vi "Navigation.vi"(0 "IA State Output in":T1, 7 "a1":dbl=10.0, 9 "a3":dbl=15.0, 11 "GoTo Navigation":bool, 12 "Debug":bool, 13 "output inc":dbl, 14 "output xy":dbl, 15 "output angle":dbl) -> (4 "IA State Output out":T1)   [LabVIEW 2017]
uses:
  Core/AI Input.ctl
  Core/AI Robot.ctl
  Intel/Functions Enum.ctl
  Intel/AttackerStates.ctl
  Path Planning/RRT/PathDests.ctl
  Path Planning/RRT/PathDest.ctl
  Core/AI Ball.ctl
  Core/Field Size.ctl
  Core/AI Judge.ctl
  Intel/Command Enum.ctl
  Util/Events/Events.ctl
panel:
  out "time 10":dbl
  out "time 9":dbl
  out "time 8":dbl
  out "time 7":dbl
  out "time 6":dbl
  out "time 5":dbl
  out "time 4":dbl
  out "time 3":dbl
  out "time 2":dbl
  out "time":dbl
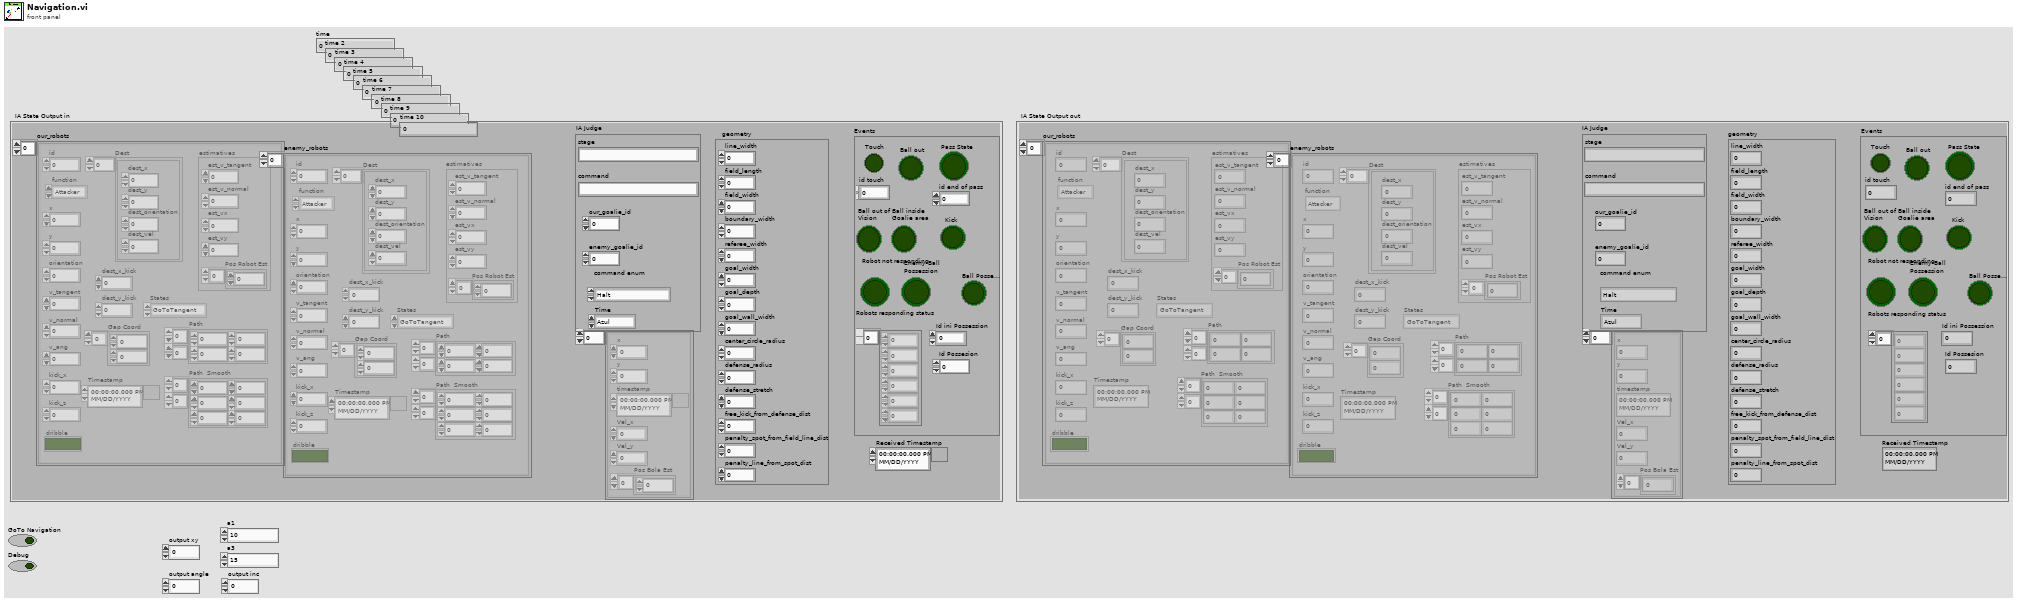
[diagram p1: front panel]
types:
  T1 = typedef "AI Input.ctl" = cluster{"our_robots":T2[], "enemy_robots":T2[], "balls":T7[], "geometry":T8, "IA Judge":T9, "Received Timestamp":timestamp, "Events":T11}
  T2 = typedef "AI Robot.ctl" = cluster{"id":u32, "function":T3, "x":dbl, "y":dbl, "orientation":dbl, "v_tangent":dbl, "v_normal":dbl, "v_ang":dbl, "kick_x":dbl, "kick_z":dbl, "dribble":bool, "Timestamp":timestamp, "estimatives":cluster{"est_v_tangent":dbl, "est_v_normal":dbl, "est_vx":dbl, "est_vy":dbl, "Pos Robot Est":dbl[]}, "dest_x_kick":dbl, "dest_y_kick":dbl, "Gap Coord":dbl[], "States":T4, "Path ":dbl[][], "Path  Smooth":dbl[][], "Dest":T5}
  T3 = typedef "Functions Enum.ctl" = enum16{"Attacker", "Goalie", "Defender", "Striker", "Goto 0", "Dummy", "Kicker", "ZigZag"}
  T4 = typedef "AttackerStates.ctl" = enum16{"Pass", "GoToTangent", "BallGetting", "GoToKick", ""}
  T5 = typedef "PathDests.ctl" = T6[]
  T6 = typedef "PathDest.ctl" = cluster{"dest_x":dbl, "dest_y":dbl, "dest_orientation":dbl, "dest_vel":dbl}
  T7 = typedef "AI Ball.ctl" = cluster{"x":dbl, "y":dbl, "timestamp":timestamp, "Vel_x":dbl, "Vel_y":dbl, "Pos Bola Est":dbl[]}
  T8 = typedef "Field Size.ctl" = cluster{"line_width":u32, "field_length":u32, "field_width":u32, "boundary_width":u32, "referee_width":u32, "goal_width":u32, "goal_depth":u32, "goal_wall_width":u32, "center_circle_radius":u32, "defense_radius":u32, "defense_stretch":u32, "free_kick_from_defense_dist":u32, "penalty_spot_from_field_line_dist":u32, "penalty_line_from_spot_dist":u32}
  T9 = typedef "AI Judge.ctl" = cluster{"stage":string, "command":string, "our_goalie_id":dbl, "enemy_goalie_id":dbl, "command enum":T10, "Time":enum16{"Azul", "Amarelo"}}
  T10 = typedef "Command Enum.ctl" = enum16{"Halt", "Stop", "Force Start", "PKA Normal Start", "Prepare Kickoff Ally", "PKE Normal Start", "Prepare Kickoff Enemy", "Prepare Penalty Ally", "PPA Normal Start", "Prepare Penalty Enemy", "PPE Normal Start", "Direct Free Enemy", "Direct Free Ally", "Indirect Free Enemy", "Indirect Free Ally", "Timeout Enemy", "Timeout Ally", "Goal Enemy", "Goal Ally", "Ball Placement Enemy", "Ball Placement Ally", "Normal Half Time", "Extra Time Break", "Extra Half Time", "None", "Post Game"}
  T11 = typedef "Events.ctl" = cluster{"Touch":bool, "Ball out":bool, "id touch":dbl, "Ball out of \nVision":bool, "Ball inside \nGoalie area":bool, "Robot not responding":bool, "Robots responding status":dbl[], "Enemy Ball \nPossession":bool, "Pass State":bool, "id end of pass":dbl, "Kick":bool, "Id ini Possession":dbl, "Ball Possesion":bool, "Id Possesion":dbl}
  T12 = cluster{"est_v_tangent":dbl, "est_v_normal":dbl, "est_vx":dbl, "est_vy":dbl, "Pos Robot Est":dbl[]}
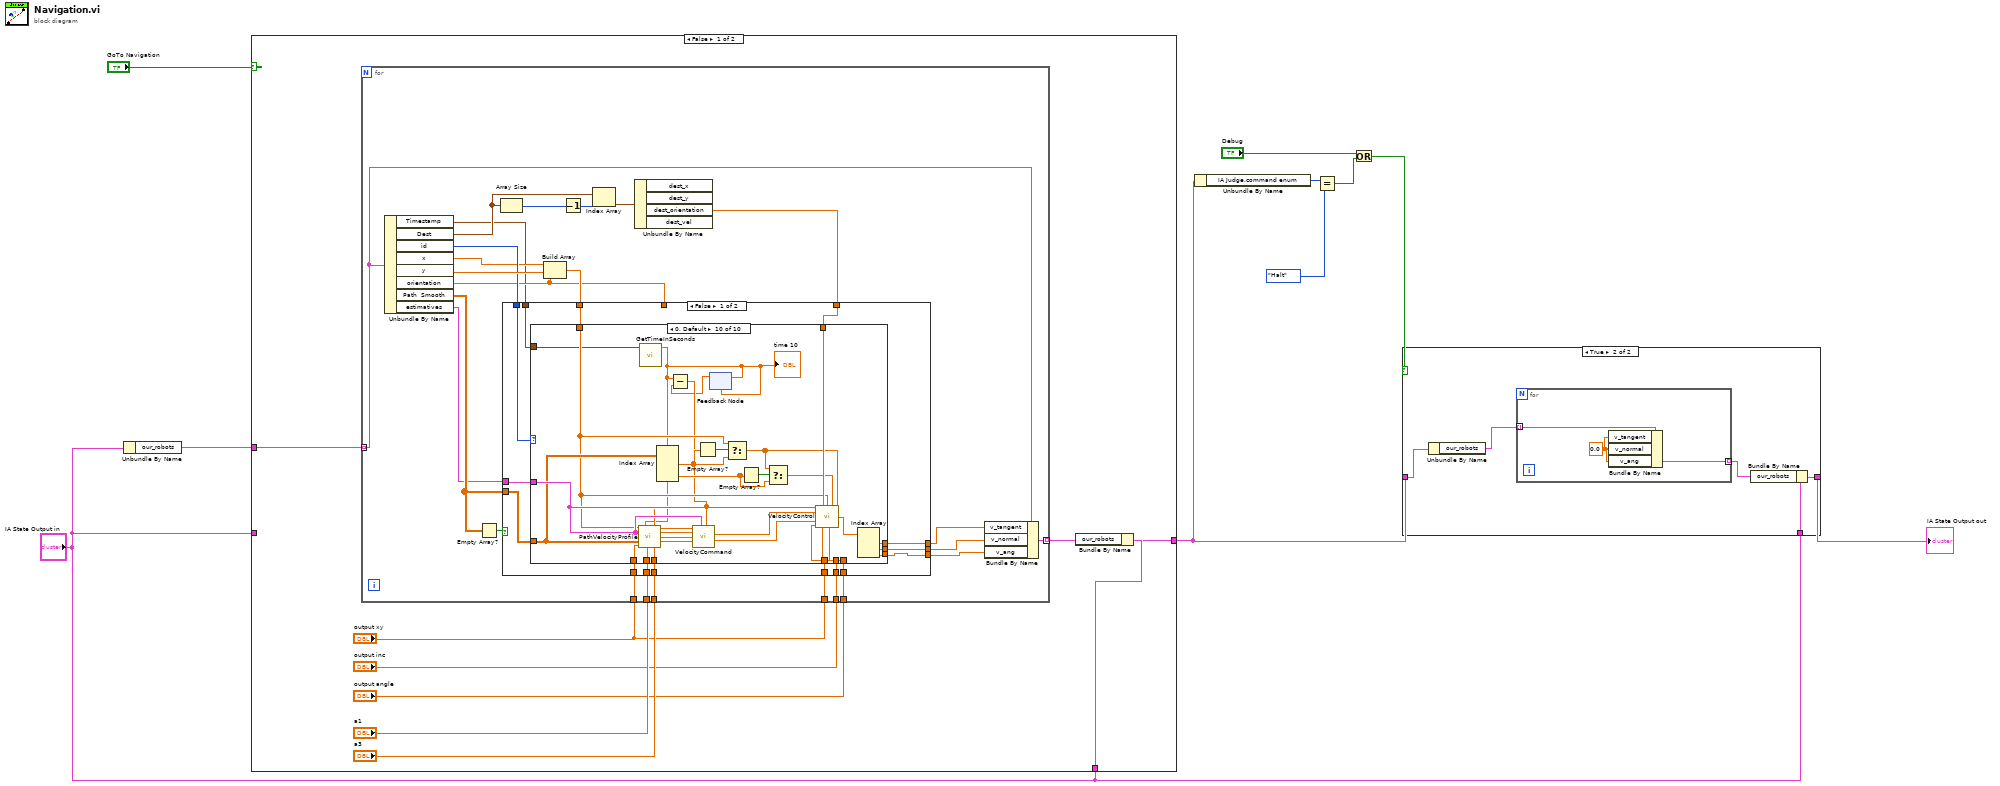
[diagram p0: block diagram]
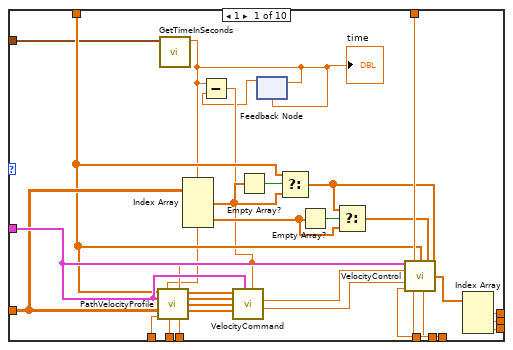
[diagram p2: hidden frame]
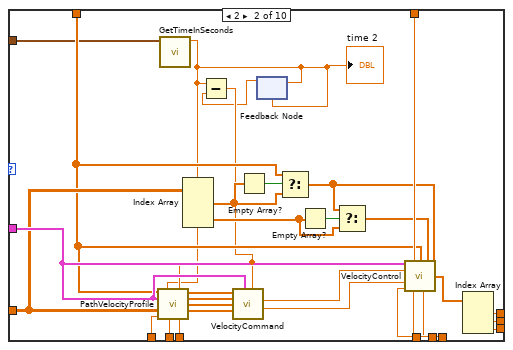
[diagram p3: hidden frame]
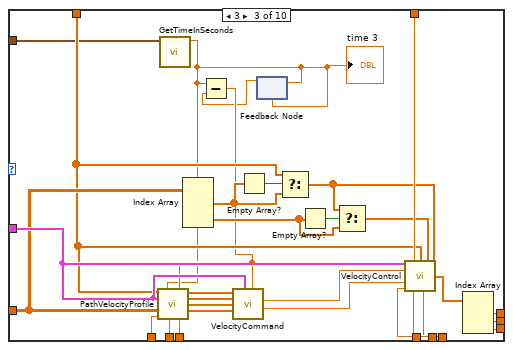
[diagram p4: hidden frame]
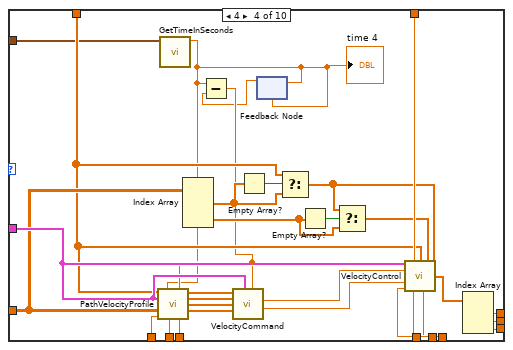
[diagram p5: hidden frame]
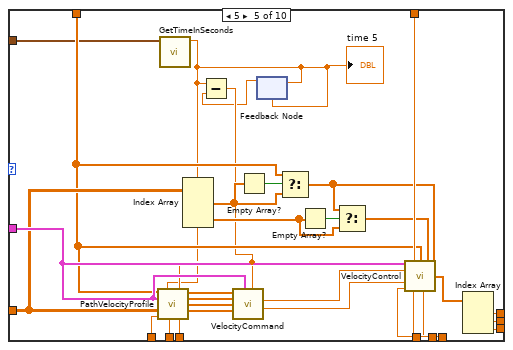
[diagram p6: hidden frame]
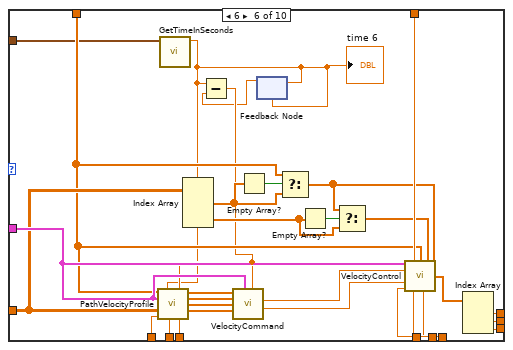
[diagram p7: hidden frame]
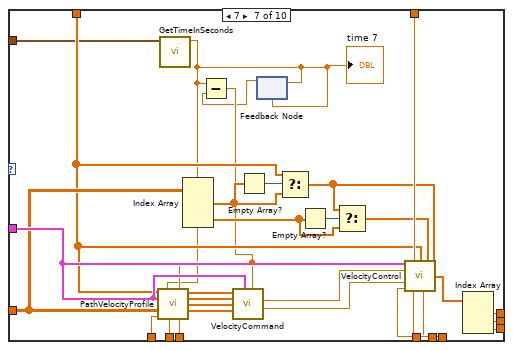
[diagram p8: hidden frame]
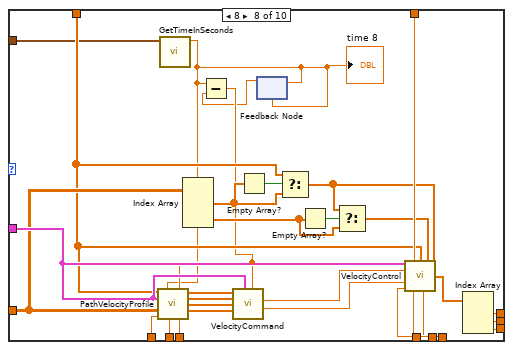
[diagram p9: hidden frame]
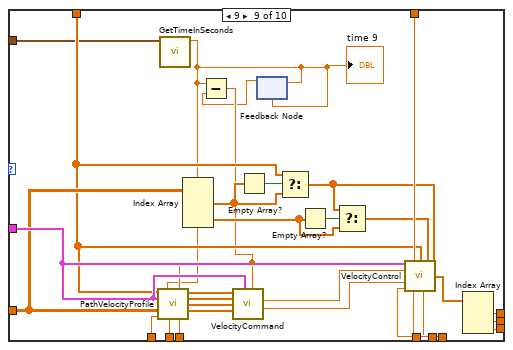
[diagram p10: hidden frame]
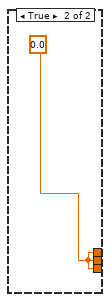
[diagram p11: hidden frame]
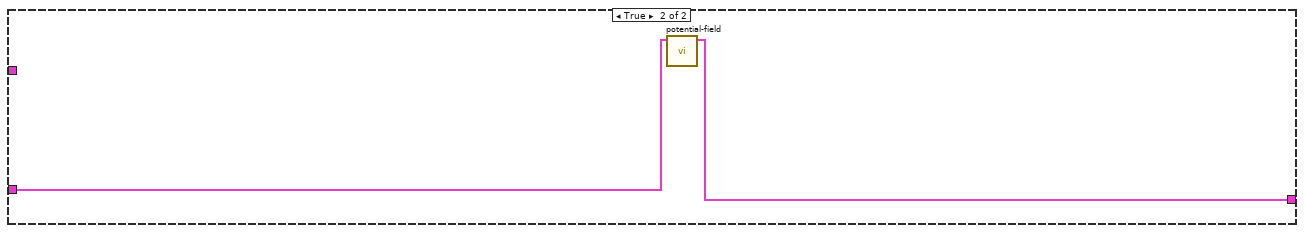
[diagram p12: hidden frame]
diagram:
  n1 = Unbundle By Name("IA State Output in") -> ("our_robots"=w10:T2[])
  n2 = case shown="False" "GoTo Navigation" {
    tunnel: w10 -> [w19 _]
    tunnel: [w16 w361] -> w6
    tunnel: "IA State Output in" -> [_ w362]
    tunnel: "IA State Output in" -> [w17 _]
    frame False {
      n3 = for {
        tunnel: w19 -> [w43] mode=indexing
        tunnel: [w42] -> w18 mode=indexing
        tunnel: "output xy" -> [w30]
        tunnel: "a1" -> [w29]
        tunnel: "a3" -> [w28]
        tunnel: "output inc" -> [w24]
        tunnel: "output angle" -> [w23]
        tunnel: "output xy" -> [w22]
        n4 = Unbundle By Name(w43) -> ("Timestamp"=w20:timestamp, "Dest"=w41:T5, "id"=w34:u32, "x"=w33:dbl, "y"=w44:dbl, "orientation"=w27:dbl, "Path  Smooth"=w35:dbl[][], "estimatives"=w31:T12)
        n5 = Empty Array?(array=w35) -> (empty?=w36:bool)
        n6 = Array Size(array=w41) -> (size(s)=w40:i32)
        n7 = Build Array(w33, w44, w27) -> (w32:dbl[])
        n8 = Decrement(x=w40) -> (x-1=w39:i32)
        n9 = Index Array(array=w41, index=w39) -> (element=w38:T6)
        n10 = Unbundle By Name(w38) -> ("dest_orientation"=w37:dbl)  [unwired: 3 out]
        n11 = case shown="False" w36 {
          tunnel: [w49 w360] -> w26
          tunnel: [w48 w360] -> w25
          tunnel: [w47 w360] -> w21
          tunnel: w34 -> [w45 _]
          tunnel: w35 -> [w51 _]
          tunnel: w37 -> [w52 _]
          tunnel: w32 -> [w50 _]
          tunnel: w31 -> [w53 _]
          tunnel: w30 -> [w59 _]
          tunnel: w29 -> [w58 _]
          tunnel: w28 -> [w57 _]
          tunnel: w27 -> [_ _]
          tunnel: w24 -> [w56 _]
          tunnel: w23 -> [w55 _]
          tunnel: w22 -> [w54 _]
          tunnel: w20 -> [w46 _]
          frame False {
            n12 = case shown="0, Default" w45 {
              tunnel: w59 -> [w89 w119 w149 w179 w209 w239 w269 w299 w329 w359]
              tunnel: w58 -> [w88 w118 w148 w178 w208 w238 w268 w298 w328 w358]
              tunnel: w57 -> [w87 w117 w147 w177 w207 w237 w267 w297 w327 w357]
              tunnel: w56 -> [w86 w116 w146 w176 w206 w236 w266 w296 w326 w356]
              tunnel: w55 -> [w85 w115 w145 w175 w205 w235 w265 w295 w325 w355]
              tunnel: w54 -> [w84 w114 w144 w174 w204 w234 w264 w294 w324 w354]
              tunnel: w53 -> [w83 w113 w143 w173 w203 w233 w263 w293 w323 w353]
              tunnel: w52 -> [w82 w112 w142 w172 w202 w232 w262 w292 w322 w352]
              tunnel: w51 -> [w81 w111 w141 w171 w201 w231 w261 w291 w321 w351]
              tunnel: w50 -> [w80 w110 w140 w170 w200 w230 w260 w290 w320 w350]
              tunnel: [w79 w109 w139 w169 w199 w229 w259 w289 w319 w349] -> w49
              tunnel: [w78 w108 w138 w168 w198 w228 w258 w288 w318 w348] -> w48
              tunnel: [w77 w107 w137 w167 w197 w227 w257 w287 w317 w347] -> w47
              tunnel: w46 -> [w63 w93 w123 w153 w183 w213 w243 w273 w303 w333]
              frame 1 {
                n13 = call "GetTimeInSeconds.vi"("Timestamp"=w63) -> ("Numeric"=w60:dbl)  [unwired: 10 in]
                "time" <- w60
                n14 = Index Array(array=w81) -> (element #1=w65:dbl[], element #2=w68:dbl[])  [unwired: 4 in]
                n15 = Empty Array?(array=w65) -> (empty?=w66:bool)
                n16 = feedback #1(w60) -> (w61:dbl)
                n17 = Subtract(x=w60, y=w61) -> (x-y=w62:dbl)
                n18 = call "PathVelocityProfile.vi"("Pose"=w80, "time"=w60, "intervalo"=w62, "estimatives"=w83, "Path  Smooth"=w81, "V_max"=w89, "Accel"=w88, "DesAccel"=w87) -> ("Time X"=w75:dbl[], "Velocities X"=w74:dbl[], "Time Y"=w73:dbl[], "Velocities Y"=w72:dbl[])  [unwired: 4 in]
                n19 = call "VelocityCommand.vi"("intervalo"=w62, "estimatives"=w83, "Velocities Y"=w72, "Time Y"=w73, "Velocities X"=w74, "Time X"=w75) -> ("Vy"=w71:dbl, "Vx"=w70:dbl)  [unwired: 4 in]
                n20 = feedback-in #1(w60) -> ()
                n21 = Select(t=w80, s=w66, f=w65) -> (s? t:f=w64:dbl[])
                n22 = Empty Array?(array=w68) -> (empty?=w69:bool)
                n23 = Select(t=w64, s=w69, f=w68) -> (s? t:f=w67:dbl[])
                n24 = call "VelocityControl.vi"("estimatives"=w83, "Dest_orientation"=w82, "Position"=w80, "Waypoint 1"=w67, "Waypoint 0"=w64, "Vx"=w70, "Vy"=w71, "output xy"=w84, "output inc"=w86, "output angle"=w85) -> ("Output Velocity"=w76:dbl[])  [unwired: 5 in]
                n25 = Index Array(array=w76) -> (element #1=w79:dbl, element #2=w78:dbl, element #3=w77:dbl)  [unwired: 3 in]
              }
              frame 2 {
                n26 = call "GetTimeInSeconds.vi"("Timestamp"=w93) -> ("Numeric"=w90:dbl)  [unwired: 10 in]
                "time 2" <- w90
                n27 = Index Array(array=w111) -> (element #1=w95:dbl[], element #2=w98:dbl[])  [unwired: 4 in]
                n28 = Empty Array?(array=w95) -> (empty?=w96:bool)
                n29 = feedback #2(w90) -> (w91:dbl)
                n30 = Subtract(x=w90, y=w91) -> (x-y=w92:dbl)
                n31 = call "PathVelocityProfile.vi"("Pose"=w110, "time"=w90, "intervalo"=w92, "estimatives"=w113, "Path  Smooth"=w111, "V_max"=w119, "Accel"=w118, "DesAccel"=w117) -> ("Time X"=w105:dbl[], "Velocities X"=w104:dbl[], "Time Y"=w103:dbl[], "Velocities Y"=w102:dbl[])  [unwired: 4 in]
                n32 = call "VelocityCommand.vi"("intervalo"=w92, "estimatives"=w113, "Velocities Y"=w102, "Time Y"=w103, "Velocities X"=w104, "Time X"=w105) -> ("Vy"=w101:dbl, "Vx"=w100:dbl)  [unwired: 4 in]
                n33 = feedback-in #2(w90) -> ()
                n34 = Select(t=w110, s=w96, f=w95) -> (s? t:f=w94:dbl[])
                n35 = Empty Array?(array=w98) -> (empty?=w99:bool)
                n36 = Select(t=w94, s=w99, f=w98) -> (s? t:f=w97:dbl[])
                n37 = call "VelocityControl.vi"("estimatives"=w113, "Dest_orientation"=w112, "Position"=w110, "Waypoint 1"=w97, "Waypoint 0"=w94, "Vx"=w100, "Vy"=w101, "output xy"=w114, "output inc"=w116, "output angle"=w115) -> ("Output Velocity"=w106:dbl[])  [unwired: 5 in]
                n38 = Index Array(array=w106) -> (element #1=w109:dbl, element #2=w108:dbl, element #3=w107:dbl)  [unwired: 3 in]
              }
              frame 3 {
                n39 = call "GetTimeInSeconds.vi"("Timestamp"=w123) -> ("Numeric"=w120:dbl)  [unwired: 10 in]
                "time 3" <- w120
                n40 = Index Array(array=w141) -> (element #1=w125:dbl[], element #2=w128:dbl[])  [unwired: 4 in]
                n41 = Empty Array?(array=w125) -> (empty?=w126:bool)
                n42 = feedback #3(w120) -> (w121:dbl)
                n43 = Subtract(x=w120, y=w121) -> (x-y=w122:dbl)
                n44 = call "PathVelocityProfile.vi"("Pose"=w140, "time"=w120, "intervalo"=w122, "estimatives"=w143, "Path  Smooth"=w141, "V_max"=w149, "Accel"=w148, "DesAccel"=w147) -> ("Time X"=w135:dbl[], "Velocities X"=w134:dbl[], "Time Y"=w133:dbl[], "Velocities Y"=w132:dbl[])  [unwired: 4 in]
                n45 = call "VelocityCommand.vi"("intervalo"=w122, "estimatives"=w143, "Velocities Y"=w132, "Time Y"=w133, "Velocities X"=w134, "Time X"=w135) -> ("Vy"=w131:dbl, "Vx"=w130:dbl)  [unwired: 4 in]
                n46 = feedback-in #3(w120) -> ()
                n47 = Select(t=w140, s=w126, f=w125) -> (s? t:f=w124:dbl[])
                n48 = Empty Array?(array=w128) -> (empty?=w129:bool)
                n49 = Select(t=w124, s=w129, f=w128) -> (s? t:f=w127:dbl[])
                n50 = call "VelocityControl.vi"("estimatives"=w143, "Dest_orientation"=w142, "Position"=w140, "Waypoint 1"=w127, "Waypoint 0"=w124, "Vx"=w130, "Vy"=w131, "output xy"=w144, "output inc"=w146, "output angle"=w145) -> ("Output Velocity"=w136:dbl[])  [unwired: 5 in]
                n51 = Index Array(array=w136) -> (element #1=w139:dbl, element #2=w138:dbl, element #3=w137:dbl)  [unwired: 3 in]
              }
              frame 4 {
                n52 = call "GetTimeInSeconds.vi"("Timestamp"=w153) -> ("Numeric"=w150:dbl)  [unwired: 10 in]
                "time 4" <- w150
                n53 = Index Array(array=w171) -> (element #1=w155:dbl[], element #2=w158:dbl[])  [unwired: 4 in]
                n54 = Empty Array?(array=w155) -> (empty?=w156:bool)
                n55 = feedback #4(w150) -> (w151:dbl)
                n56 = Subtract(x=w150, y=w151) -> (x-y=w152:dbl)
                n57 = call "PathVelocityProfile.vi"("Pose"=w170, "time"=w150, "intervalo"=w152, "estimatives"=w173, "Path  Smooth"=w171, "V_max"=w179, "Accel"=w178, "DesAccel"=w177) -> ("Time X"=w165:dbl[], "Velocities X"=w164:dbl[], "Time Y"=w163:dbl[], "Velocities Y"=w162:dbl[])  [unwired: 4 in]
                n58 = call "VelocityCommand.vi"("intervalo"=w152, "estimatives"=w173, "Velocities Y"=w162, "Time Y"=w163, "Velocities X"=w164, "Time X"=w165) -> ("Vy"=w161:dbl, "Vx"=w160:dbl)  [unwired: 4 in]
                n59 = feedback-in #4(w150) -> ()
                n60 = Select(t=w170, s=w156, f=w155) -> (s? t:f=w154:dbl[])
                n61 = Empty Array?(array=w158) -> (empty?=w159:bool)
                n62 = Select(t=w154, s=w159, f=w158) -> (s? t:f=w157:dbl[])
                n63 = call "VelocityControl.vi"("estimatives"=w173, "Dest_orientation"=w172, "Position"=w170, "Waypoint 1"=w157, "Waypoint 0"=w154, "Vx"=w160, "Vy"=w161, "output xy"=w174, "output inc"=w176, "output angle"=w175) -> ("Output Velocity"=w166:dbl[])  [unwired: 5 in]
                n64 = Index Array(array=w166) -> (element #1=w169:dbl, element #2=w168:dbl, element #3=w167:dbl)  [unwired: 3 in]
              }
              frame 5 {
                n65 = call "GetTimeInSeconds.vi"("Timestamp"=w183) -> ("Numeric"=w180:dbl)  [unwired: 10 in]
                "time 5" <- w180
                n66 = Index Array(array=w201) -> (element #1=w185:dbl[], element #2=w188:dbl[])  [unwired: 4 in]
                n67 = Empty Array?(array=w185) -> (empty?=w186:bool)
                n68 = feedback #5(w180) -> (w181:dbl)
                n69 = Subtract(x=w180, y=w181) -> (x-y=w182:dbl)
                n70 = call "PathVelocityProfile.vi"("Pose"=w200, "time"=w180, "intervalo"=w182, "estimatives"=w203, "Path  Smooth"=w201, "V_max"=w209, "Accel"=w208, "DesAccel"=w207) -> ("Time X"=w195:dbl[], "Velocities X"=w194:dbl[], "Time Y"=w193:dbl[], "Velocities Y"=w192:dbl[])  [unwired: 4 in]
                n71 = call "VelocityCommand.vi"("intervalo"=w182, "estimatives"=w203, "Velocities Y"=w192, "Time Y"=w193, "Velocities X"=w194, "Time X"=w195) -> ("Vy"=w191:dbl, "Vx"=w190:dbl)  [unwired: 4 in]
                n72 = feedback-in #5(w180) -> ()
                n73 = Select(t=w200, s=w186, f=w185) -> (s? t:f=w184:dbl[])
                n74 = Empty Array?(array=w188) -> (empty?=w189:bool)
                n75 = Select(t=w184, s=w189, f=w188) -> (s? t:f=w187:dbl[])
                n76 = call "VelocityControl.vi"("estimatives"=w203, "Dest_orientation"=w202, "Position"=w200, "Waypoint 1"=w187, "Waypoint 0"=w184, "Vx"=w190, "Vy"=w191, "output xy"=w204, "output inc"=w206, "output angle"=w205) -> ("Output Velocity"=w196:dbl[])  [unwired: 5 in]
                n77 = Index Array(array=w196) -> (element #1=w199:dbl, element #2=w198:dbl, element #3=w197:dbl)  [unwired: 3 in]
              }
              frame 6 {
                n78 = call "GetTimeInSeconds.vi"("Timestamp"=w213) -> ("Numeric"=w210:dbl)  [unwired: 10 in]
                "time 6" <- w210
                n79 = Index Array(array=w231) -> (element #1=w215:dbl[], element #2=w218:dbl[])  [unwired: 4 in]
                n80 = Empty Array?(array=w215) -> (empty?=w216:bool)
                n81 = feedback #6(w210) -> (w211:dbl)
                n82 = Subtract(x=w210, y=w211) -> (x-y=w212:dbl)
                n83 = call "PathVelocityProfile.vi"("Pose"=w230, "time"=w210, "intervalo"=w212, "estimatives"=w233, "Path  Smooth"=w231, "V_max"=w239, "Accel"=w238, "DesAccel"=w237) -> ("Time X"=w225:dbl[], "Velocities X"=w224:dbl[], "Time Y"=w223:dbl[], "Velocities Y"=w222:dbl[])  [unwired: 4 in]
                n84 = call "VelocityCommand.vi"("intervalo"=w212, "estimatives"=w233, "Velocities Y"=w222, "Time Y"=w223, "Velocities X"=w224, "Time X"=w225) -> ("Vy"=w221:dbl, "Vx"=w220:dbl)  [unwired: 4 in]
                n85 = feedback-in #6(w210) -> ()
                n86 = Select(t=w230, s=w216, f=w215) -> (s? t:f=w214:dbl[])
                n87 = Empty Array?(array=w218) -> (empty?=w219:bool)
                n88 = Select(t=w214, s=w219, f=w218) -> (s? t:f=w217:dbl[])
                n89 = call "VelocityControl.vi"("estimatives"=w233, "Dest_orientation"=w232, "Position"=w230, "Waypoint 1"=w217, "Waypoint 0"=w214, "Vx"=w220, "Vy"=w221, "output xy"=w234, "output inc"=w236, "output angle"=w235) -> ("Output Velocity"=w226:dbl[])  [unwired: 5 in]
                n90 = Index Array(array=w226) -> (element #1=w229:dbl, element #2=w228:dbl, element #3=w227:dbl)  [unwired: 3 in]
              }
              frame 7 {
                n91 = call "GetTimeInSeconds.vi"("Timestamp"=w243) -> ("Numeric"=w240:dbl)  [unwired: 10 in]
                "time 7" <- w240
                n92 = Index Array(array=w261) -> (element #1=w245:dbl[], element #2=w248:dbl[])  [unwired: 4 in]
                n93 = Empty Array?(array=w245) -> (empty?=w246:bool)
                n94 = feedback #7(w240) -> (w241:dbl)
                n95 = Subtract(x=w240, y=w241) -> (x-y=w242:dbl)
                n96 = call "PathVelocityProfile.vi"("Pose"=w260, "time"=w240, "intervalo"=w242, "estimatives"=w263, "Path  Smooth"=w261, "V_max"=w269, "Accel"=w268, "DesAccel"=w267) -> ("Time X"=w255:dbl[], "Velocities X"=w254:dbl[], "Time Y"=w253:dbl[], "Velocities Y"=w252:dbl[])  [unwired: 4 in]
                n97 = call "VelocityCommand.vi"("intervalo"=w242, "estimatives"=w263, "Velocities Y"=w252, "Time Y"=w253, "Velocities X"=w254, "Time X"=w255) -> ("Vy"=w251:dbl, "Vx"=w250:dbl)  [unwired: 4 in]
                n98 = feedback-in #7(w240) -> ()
                n99 = Select(t=w260, s=w246, f=w245) -> (s? t:f=w244:dbl[])
                n100 = Empty Array?(array=w248) -> (empty?=w249:bool)
                n101 = Select(t=w244, s=w249, f=w248) -> (s? t:f=w247:dbl[])
                n102 = call "VelocityControl.vi"("estimatives"=w263, "Dest_orientation"=w262, "Position"=w260, "Waypoint 1"=w247, "Waypoint 0"=w244, "Vx"=w250, "Vy"=w251, "output xy"=w264, "output inc"=w266, "output angle"=w265) -> ("Output Velocity"=w256:dbl[])  [unwired: 5 in]
                n103 = Index Array(array=w256) -> (element #1=w259:dbl, element #2=w258:dbl, element #3=w257:dbl)  [unwired: 3 in]
              }
              frame 8 {
                n104 = call "GetTimeInSeconds.vi"("Timestamp"=w273) -> ("Numeric"=w270:dbl)  [unwired: 10 in]
                "time 8" <- w270
                n105 = Index Array(array=w291) -> (element #1=w275:dbl[], element #2=w278:dbl[])  [unwired: 4 in]
                n106 = Empty Array?(array=w275) -> (empty?=w276:bool)
                n107 = feedback #8(w270) -> (w271:dbl)
                n108 = Subtract(x=w270, y=w271) -> (x-y=w272:dbl)
                n109 = call "PathVelocityProfile.vi"("Pose"=w290, "time"=w270, "intervalo"=w272, "estimatives"=w293, "Path  Smooth"=w291, "V_max"=w299, "Accel"=w298, "DesAccel"=w297) -> ("Time X"=w285:dbl[], "Velocities X"=w284:dbl[], "Time Y"=w283:dbl[], "Velocities Y"=w282:dbl[])  [unwired: 4 in]
                n110 = call "VelocityCommand.vi"("intervalo"=w272, "estimatives"=w293, "Velocities Y"=w282, "Time Y"=w283, "Velocities X"=w284, "Time X"=w285) -> ("Vy"=w281:dbl, "Vx"=w280:dbl)  [unwired: 4 in]
                n111 = feedback-in #8(w270) -> ()
                n112 = Select(t=w290, s=w276, f=w275) -> (s? t:f=w274:dbl[])
                n113 = Empty Array?(array=w278) -> (empty?=w279:bool)
                n114 = Select(t=w274, s=w279, f=w278) -> (s? t:f=w277:dbl[])
                n115 = call "VelocityControl.vi"("estimatives"=w293, "Dest_orientation"=w292, "Position"=w290, "Waypoint 1"=w277, "Waypoint 0"=w274, "Vx"=w280, "Vy"=w281, "output xy"=w294, "output inc"=w296, "output angle"=w295) -> ("Output Velocity"=w286:dbl[])  [unwired: 5 in]
                n116 = Index Array(array=w286) -> (element #1=w289:dbl, element #2=w288:dbl, element #3=w287:dbl)  [unwired: 3 in]
              }
              frame 9 {
                n117 = call "GetTimeInSeconds.vi"("Timestamp"=w303) -> ("Numeric"=w300:dbl)  [unwired: 10 in]
                "time 9" <- w300
                n118 = Index Array(array=w321) -> (element #1=w305:dbl[], element #2=w308:dbl[])  [unwired: 4 in]
                n119 = Empty Array?(array=w305) -> (empty?=w306:bool)
                n120 = feedback #9(w300) -> (w301:dbl)
                n121 = Subtract(x=w300, y=w301) -> (x-y=w302:dbl)
                n122 = call "PathVelocityProfile.vi"("Pose"=w320, "time"=w300, "intervalo"=w302, "estimatives"=w323, "Path  Smooth"=w321, "V_max"=w329, "Accel"=w328, "DesAccel"=w327) -> ("Time X"=w315:dbl[], "Velocities X"=w314:dbl[], "Time Y"=w313:dbl[], "Velocities Y"=w312:dbl[])  [unwired: 4 in]
                n123 = call "VelocityCommand.vi"("intervalo"=w302, "estimatives"=w323, "Velocities Y"=w312, "Time Y"=w313, "Velocities X"=w314, "Time X"=w315) -> ("Vy"=w311:dbl, "Vx"=w310:dbl)  [unwired: 4 in]
                n124 = feedback-in #9(w300) -> ()
                n125 = Select(t=w320, s=w306, f=w305) -> (s? t:f=w304:dbl[])
                n126 = Empty Array?(array=w308) -> (empty?=w309:bool)
                n127 = Select(t=w304, s=w309, f=w308) -> (s? t:f=w307:dbl[])
                n128 = call "VelocityControl.vi"("estimatives"=w323, "Dest_orientation"=w322, "Position"=w320, "Waypoint 1"=w307, "Waypoint 0"=w304, "Vx"=w310, "Vy"=w311, "output xy"=w324, "output inc"=w326, "output angle"=w325) -> ("Output Velocity"=w316:dbl[])  [unwired: 5 in]
                n129 = Index Array(array=w316) -> (element #1=w319:dbl, element #2=w318:dbl, element #3=w317:dbl)  [unwired: 3 in]
              }
              frame 0, Default {
                n130 = call "GetTimeInSeconds.vi"("Timestamp"=w333) -> ("Numeric"=w330:dbl)  [unwired: 10 in]
                "time 10" <- w330
                n131 = Index Array(array=w351) -> (element #1=w335:dbl[], element #2=w338:dbl[])  [unwired: 4 in]
                n132 = Empty Array?(array=w335) -> (empty?=w336:bool)
                n133 = feedback #10(w330) -> (w331:dbl)
                n134 = Subtract(x=w330, y=w331) -> (x-y=w332:dbl)
                n135 = call "PathVelocityProfile.vi"("Pose"=w350, "time"=w330, "intervalo"=w332, "estimatives"=w353, "Path  Smooth"=w351, "V_max"=w359, "Accel"=w358, "DesAccel"=w357) -> ("Time X"=w345:dbl[], "Velocities X"=w344:dbl[], "Time Y"=w343:dbl[], "Velocities Y"=w342:dbl[])  [unwired: 4 in]
                n136 = call "VelocityCommand.vi"("intervalo"=w332, "estimatives"=w353, "Velocities Y"=w342, "Time Y"=w343, "Velocities X"=w344, "Time X"=w345) -> ("Vy"=w341:dbl, "Vx"=w340:dbl)  [unwired: 4 in]
                n137 = feedback-in #10(w330) -> ()
                n138 = Select(t=w350, s=w336, f=w335) -> (s? t:f=w334:dbl[])
                n139 = Empty Array?(array=w338) -> (empty?=w339:bool)
                n140 = Select(t=w334, s=w339, f=w338) -> (s? t:f=w337:dbl[])
                n141 = call "VelocityControl.vi"("estimatives"=w353, "Dest_orientation"=w352, "Position"=w350, "Waypoint 1"=w337, "Waypoint 0"=w334, "Vx"=w340, "Vy"=w341, "output xy"=w354, "output inc"=w356, "output angle"=w355) -> ("Output Velocity"=w346:dbl[])  [unwired: 5 in]
                n142 = Index Array(array=w346) -> (element #1=w349:dbl, element #2=w348:dbl, element #3=w347:dbl)  [unwired: 3 in]
              }
            }
          }
          frame True {
            w360 = 0.0 ("output")
          }
        }
        n143 = Bundle By Name(cluster=w43, "v_tangent"=w26, "v_normal"=w25, "v_ang"=w21) -> (w42:T2)
      }
      n144 = Bundle By Name(cluster=w17, "our_robots"=w18) -> (w16:T1)
    }
    frame True {
      n145 = call "potential-field.vi"("IA State Output in"=w362) -> ("IA State Output out"=w361:T1)  [unwired: 10 in]
    }
  }
  n146 = Unbundle By Name(w6) -> ("IA Judge.command enum"=w5:T10)
  n147 = Equal?(x=w5, y=Command_Enum."Halt") -> (x = y?=w2:bool)
  n148 = Or(x="Debug", y=w2) -> (x .or. y?=w3:bool)
  n149 = case shown="True" w3 {
    tunnel: [w363 w368] -> w8
    tunnel: w6 -> [w363 w365]
    tunnel: "IA State Output in" -> [_ w366]
    frame False {
    }
    frame True {
      n150 = Unbundle By Name(w365) -> ("our_robots"=w364:T2[])
      n151 = for {
        tunnel: [w371] -> w367 mode=indexing
        tunnel: w364 -> [w369] mode=indexing
        w370 = 0.0 ("v_normal")
        n152 = Bundle By Name(cluster=w369, "v_tangent"=w370, "v_normal"=w370, "v_ang"=w370) -> (w371:T2)
      }
      n153 = Bundle By Name(cluster=w366, "our_robots"=w367) -> (w368:T1)
    }
  }
  "IA State Output out" <- w8
